vi "ModifyProjectDeployLVAddons.vi"() -> ()   [LabVIEW 2021]
uses:
  <vilib>/Wiresmith Technology/G CLI/CLI Class/CLI.lvclass
panel:
  out "Custom Parameters":string[](array[string])
  out "error out":errorcluster
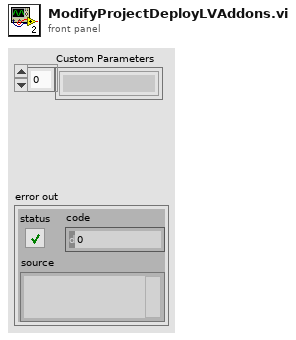
[diagram p1: front panel]
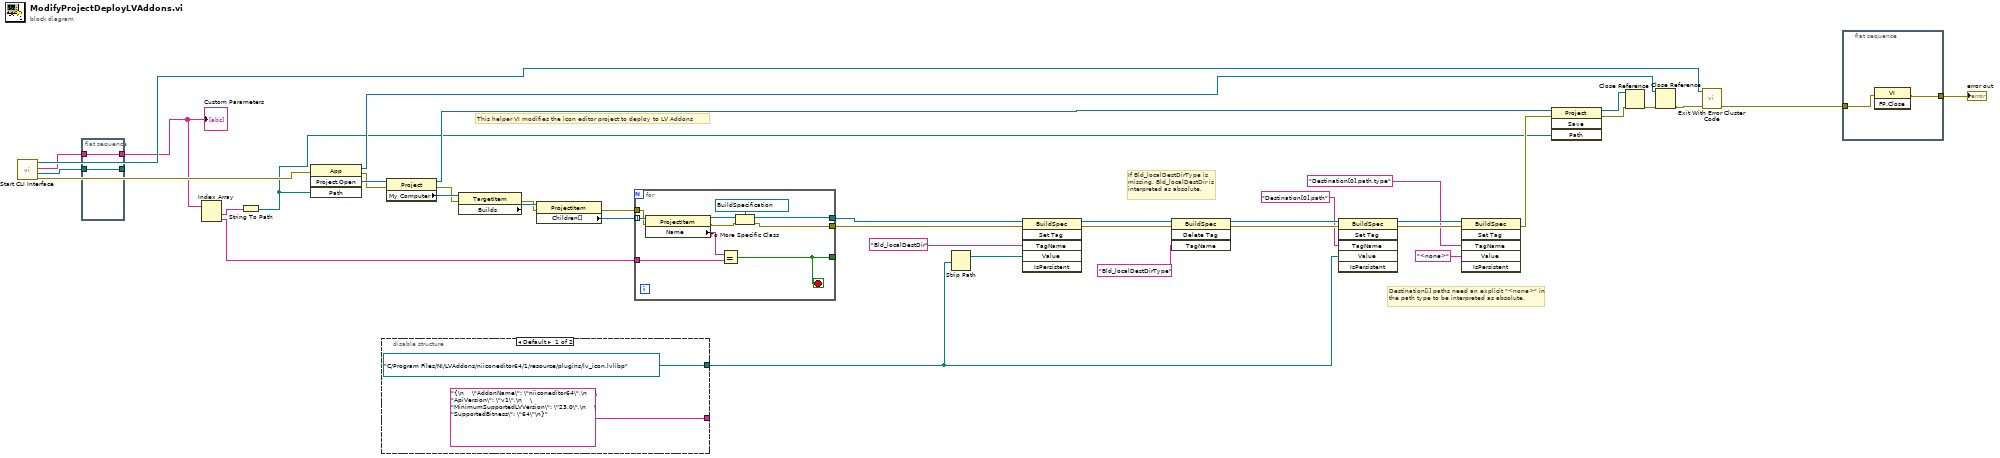
[diagram p0: block diagram]
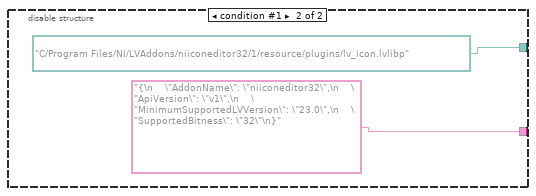
[diagram p2: hidden frame]
diagram:
  # "Destination[i] paths need an explicit \"<none>\" in the path type to be interpreted as absolute."
  # "If Bld_localDestDirType is missing, Bld_localDestDir is interpreted as absolute."
  # "This helper VI modifies the icon editor project to deploy to LV Addons"
  n1 = call <vilib>:"Start CLI Interface.vi"() -> ("error out"=w11:errorcluster, "Working Directory"=w6:path, "Custom Parameters"=w5:string[], "CLI out"=w9:refnum<class "CLI.lvclass">)  [unwired: 8 in]
  n2 = flat-sequence {
    tunnel: w6 -> [w42]
    tunnel: [w42] -> _
    tunnel: w5 -> [w41]
    tunnel: [w41] -> w4
    frame #0 {
    }
  }
  n3 = Index Array(array=w4) -> (element #1=w3:string, element #2=w1:string)  [unwired: 2 in]
  n4 = String To Path(string=w3) -> (path=w2:path)
  n5 = invoke class="App" method="Project.Open"(error in=w11, "Path"=w2) -> (reference out=w12:refnum<vi>, error out=w20:errorcluster, "Project:Open"=w35:refnum<vi>)  [unwired: 2 in, 1 out]
  n6 = disable-structure shown="Default" {
    disable-tunnel: [path "C:/Program Files/NI/LVAddons/niiconeditor64/1/resource/plugins/lv_icon.lvlibp" ("Destination[i] Paths (Absolute)") path "C:/Program Files/NI/LVAddons/niiconeditor32/1/resource/plugins/lv_icon.lvlibp" ("Destination[i] Paths (Absolute)")] -> w17
    disable-tunnel: ["{\n    \"AddonName\": \"niiconeditor64\",\n    \"ApiVersion\": \"v1\",\n    \"MinimumSupportedLVVersion\": \"23.0\",\n    \"SupportedBitness\": \"64\"\n}" ("Tag Name") "{\n    \"AddonName\": \"niiconeditor32\",\n    \"ApiVersion\": \"v1\",\n    \"MinimumSupportedLVVersion\": \"23.0\",\n    \"SupportedBitness\": \"32\"\n}" ("Tag Name")] -> _
    frame condition #0 (active) {
    }
    frame condition #1 {
    }
  }
  n7 = property class="Project"(reference=w35, error in=w20) -> (reference out=w34:refnum<vi>, error out=w19:errorcluster, "My Computer"=w40:refnum<vi>)
  n8 = property class="TargetItem"(reference=w40, error in=w19) -> (error out=w18:errorcluster, "Builds"=w38:refnum<vi>)  [unwired: 1 out]
  n9 = property class="ProjectItem"(reference=w38, error in=w18) -> (error out=w16:errorcluster, "Children[]"=w39:refnum<vi>[])  [unwired: 1 out]
  n10 = for {
    tunnel: w39 -> [w56] mode=indexing
    tunnel: [w49] -> w37
    tunnel: w1 -> [w54]
    tunnel: [w53] -> _
    tunnel: [w50] -> w36
    tunnel: w16 -> [w47]
    stop <- w53 stop-if-true
    n11 = property class="ProjectItem"(reference=w56, error in=w47) -> (reference out=w51:refnum<vi>, error out=w52:errorcluster, "Name"=w55:string)
    n12 = Equal?(x=w55, y=w54) -> (x = y?=w53:bool)
    n13 = To More Specific Class(target class=refnum<vi> refnum ("Build Spec"), reference=w51, error in=w52) -> (specific class reference=w49:refnum<vi>, error out=w50:errorcluster)
  }
  n14 = Strip Path(path=w17) -> (stripped path=w21:path)  [unwired: 1 out]
  n15 = invoke class="BuildSpec" method="Set Tag"(reference=w37, error in=w36, "TagName"="Bld_localDestDir" ("Tag Name"), "Value"=w21) -> (reference out=w33:refnum<vi>, error out=w29:errorcluster)  [unwired: 2 in, 4 out]
  n16 = invoke class="BuildSpec" method="Delete Tag"(reference=w33, error in=w29, "TagName"="Bld_localDestDirType" ("Tag Name")) -> (reference out=w32:refnum<vi>, error out=w28:errorcluster)  [unwired: 1 in, 2 out]
  n17 = invoke class="BuildSpec" method="Set Tag"(reference=w32, error in=w28, "TagName"="Destination[0].path" ("format string"), "Value"=w17) -> (reference out=w27:refnum<vi>, error out=w26:errorcluster)  [unwired: 2 in, 4 out]
  n18 = invoke class="BuildSpec" method="Set Tag"(reference=w27, error in=w26, "TagName"="Destination[0].path.type" ("format string"), "Value"="<none>") -> (error out=w22:errorcluster)  [unwired: 2 in, 5 out]
  n19 = invoke class="Project" method="Save"(reference=w34, error in=w22, "Path"=w2) -> (reference out=w14:refnum<vi>, error out=w15:errorcluster)  [unwired: 1 in, 2 out]
  n20 = Close Reference(reference=w14, error in (no error)=w15) -> (error out=w13:errorcluster)
  n21 = Close Reference(reference=w12, error in (no error)=w13) -> (error out=w10:errorcluster)
  n22 = call <vilib>:"Exit With Error Cluster Code.vi"("error in (no error)"=w10, "CLI in"=w9) -> ("error out"=w8:errorcluster)  [unwired: 9 in]
  n23 = flat-sequence {
    tunnel: [w58] -> w7
    tunnel: w8 -> [w57]
    frame #0 {
      n24 = invoke class="VI" method="FP.Close"(error in=w57) -> (error out=w58:errorcluster)  [unwired: 2 in, 2 out]
    }
  }
  "error out" <- w7
  "Custom Parameters" <- w4
